vi "sub_cmdn_fgv.vi"(7 "cmd":enum16{"ini", "a+1", "episode+1", "read"}(ring)) -> (0 "episode_str":string, 1 "count_episode":i32, 2 "action_str":string, 3 "count_action":i32)   [LabVIEW 2018]
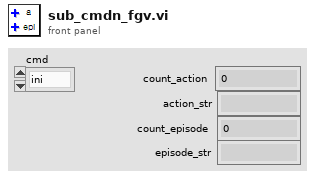
[diagram p1: front panel]
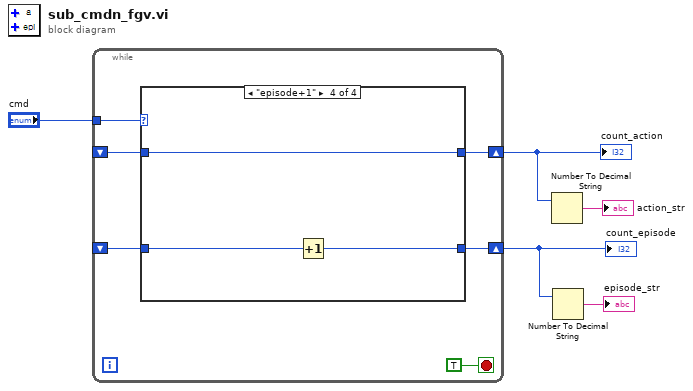
[diagram p0: block diagram]
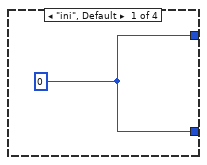
[diagram p2: hidden frame]
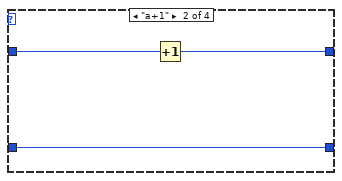
[diagram p3: hidden frame]
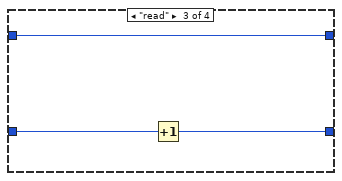
[diagram p4: hidden frame]
diagram:
  n1 = while {
    tunnel: "cmd" -> [w10]
    shift-right: [w9] -> w4
    shift-left: _ -> [w8]
    shift-right: [w7] -> w1
    shift-left: _ -> [w6]
    stop <- TRUE stop-if-true
    n2 = case shown="\"episode+1\"" w10 {
      tunnel: [w12 w14 w18 w21] -> w9
      tunnel: w8 -> [_ w15 w18 w21]
      tunnel: [w12 w13 w16 w19] -> w7
      tunnel: w6 -> [_ w13 w17 w20]
      frame "ini", Default {
        w12 = 0
      }
      frame "a+1" {
        n3 = Increment(x=w15) -> (x+1=w14:i32)
      }
      frame "read" {
        n4 = Increment(x=w17) -> (x+1=w16:i32)
      }
      frame "episode+1" {
        n5 = Increment(x=w20) -> (x+1=w19:i32)
      }
    }
  }
  "count_action" <- w4
  "count_episode" <- w1
  n6 = Number To Decimal String(number=w4) -> (decimal integer string=→"action_str":string)  [unwired: 1 in]
  n7 = Number To Decimal String(number=w1) -> (decimal integer string=→"episode_str":string)  [unwired: 1 in]
